vi "exercise4.vi"() -> ()   [LabVIEW 2020]
uses:
  <vilib>/measure/NI_MABase.lvlib
panel:
  in  "Enter amount of iterations":i32 min=0 max=250 step=1
  out "Waveform Graph":waveform(dbl)(graph)
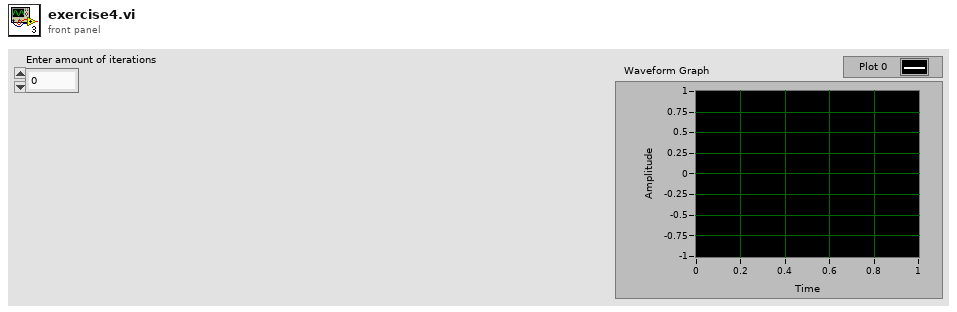
[diagram p1: front panel]
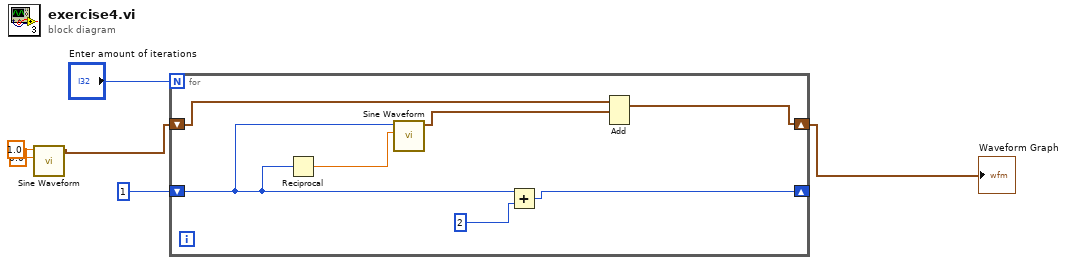
[diagram p0: block diagram]
diagram:
  n1 = call <vilib>:"Sine Waveform.vi"("amplitude"=0.0, "frequency"=1.0) -> ("signal out"=w3:waveform(dbl))  [unwired: 8 in, 1 out]
  n2 = for {
    N: "Enter amount of iterations" -> [_]
    shift-right: [w12] -> _
    shift-left: 1 -> [w7]
    shift-right: [w10] -> w4
    shift-left: w3 -> [w11]
    n3 = Reciprocal(x=w7) -> (1/x=w8:dbl)
    n4 = call <vilib>:"Sine Waveform.vi"("amplitude"=w8, "frequency"=w7) -> ("signal out"=w9:waveform(dbl))  [unwired: 8 in, 1 out]
    n5 = Add(x=w7, y=2) -> (x+y=w12:i32)
    n6 = Add(1:w9, 2:w11) -> (0:w10:waveform(dbl))  [unwired: 1 in, 1 out]
  }
  "Waveform Graph" <- w4
